vi "dfd_Render Function.vi"(0 "picture":picture, 1 "numer of element":i32=1, 3 "rect in":T1, 4 "alignment(left, top)":T2, 6 "bracket":cluster{"left":string, "right":string}={"left"="(", "right"=")"}, 7 "function name":string="y", 8 "fonts input":T3(array[cluster]), 9 "dot":bool, 11 "variable":string="n", 13 "modification":string) -> (14 "new picture":picture, 17 "rect out":T1)   [LabVIEW 2017, in "NI_DigFilter_Process.lvlib"]
uses:
  <vilib>/addons/Digital Filter Design/NI_DigFilter_Process.lvlib
panel:
  in  "Desired font(User-specified Font)":T4(ring)
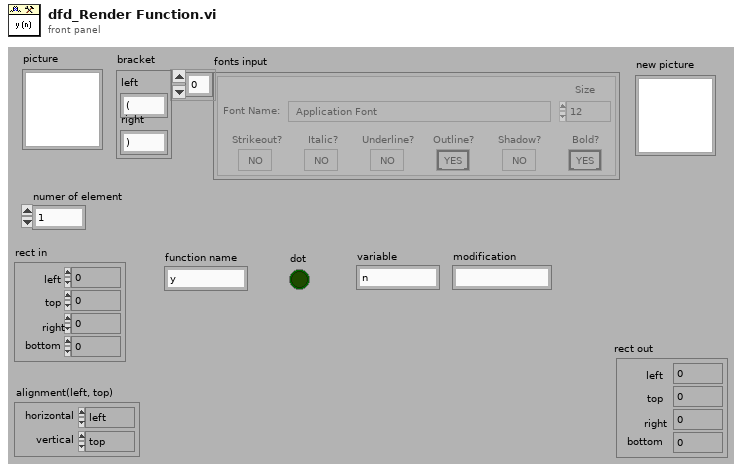
[diagram p1: front panel]
types:
  T1 = cluster{"left":i16, "top":i16, "right":i16, "bottom":i16}
  T2 = cluster{"horizontal":enum16{"left", "center", "right"}, "vertical":enum16{"top", "center", "bottom"}}
  T3 = cluster{"Font Name:":string, "Size":i16, "Strikeout?":bool, "Italic?":bool, "Underline?":bool, "Outline?":bool, "Shadow?":bool, "Bold?":bool}[]
  T4 = enum16{"User-specified Font", "Application Font", "System Font", "Dialog Font"}
  T5 = cluster{"Font Name:":string, "Size":i16, "Strikeout?":bool, "Italic?":bool, "Underline?":bool, "Outline?":bool, "Shadow?":bool, "Bold?":bool}
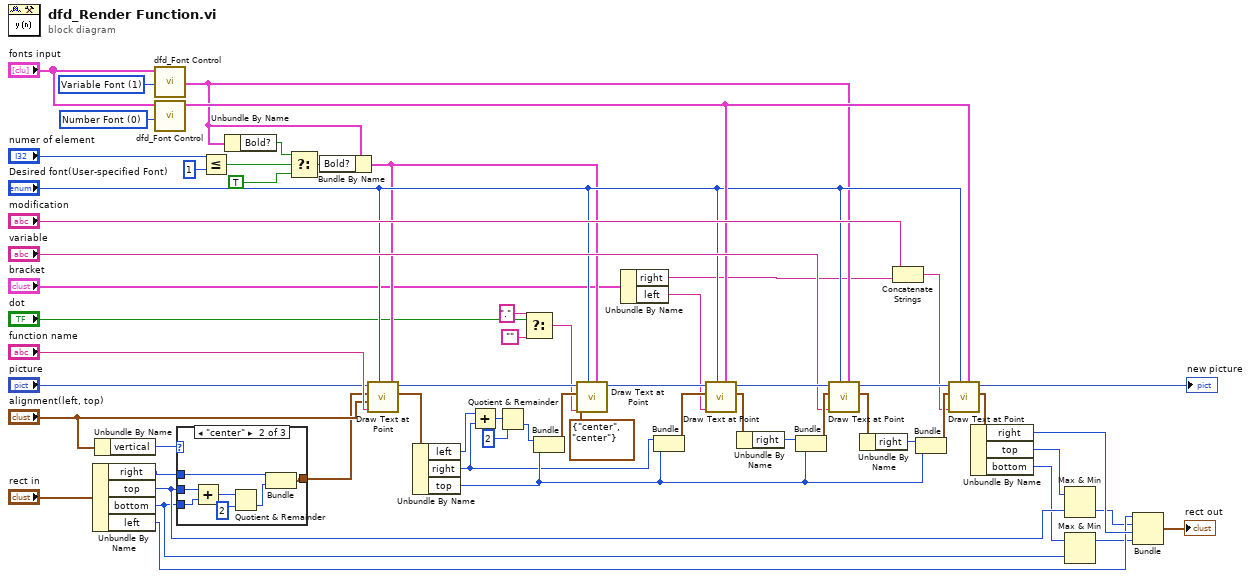
[diagram p0: block diagram]
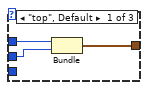
[diagram p2: hidden frame]
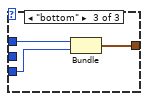
[diagram p3: hidden frame]
diagram:
  w33 = u16 1 items=["Number Font", "Variable Font", "Script Font"] ("Tpye")
  w42 = u16 0 items=["Number Font", "Variable Font", "Script Font"] ("Tpye")
  n1 = Unbundle By Name("rect in") -> ("right"=w16:i16, "top"=w12:i16, "bottom"=w5:i16, "left"=w14:i16)
  n2 = Unbundle By Name("alignment(left, top)") -> ("vertical"=w18:enum16{"top", "center", "bottom"})
  n3 = call <vilib>:"dfd_Font Control.vi"("tpye"=w33, "fonts input"="fonts input") -> ("font output"=w28:T5)  [unwired: 9 out]
  n4 = call <vilib>:"dfd_Font Control.vi"("tpye"=w42, "fonts input"="fonts input") -> ("font output"=w44:T5)  [unwired: 9 out]
  n5 = case shown="\"center\"" w18 {
    tunnel: w12 -> [w63 w70 _]
    tunnel: w16 -> [w64 w67 w74]
    tunnel: [w62 w65 w72] -> w15
    tunnel: w5 -> [_ w71 w73]
    frame "top", Default {
      n6 = Bundle("right"=w64, "top"=w63) -> (w62:cluster{"right":i16, "top":i16})  [unwired: 1 out]
    }
    frame "center" {
      n7 = Add(x=w70, y=w71) -> (x+y=w69:i16)
      n8 = Quotient & Remainder(x=w69, y=i16 2) -> (floor(x/y)=w66:i16)  [unwired: 1 out]
      n9 = Bundle("right"=w67, w66) -> (w65:cluster{"right":i16, i16})  [unwired: 1 out]
    }
    frame "bottom" {
      n10 = Bundle("right"=w74, "bottom"=w73) -> (w72:cluster{"right":i16, "bottom":i16})  [unwired: 1 out]
    }
  }
  n11 = Less Or Equal?(x="numer of element", y=1) -> (x <= y?=w41:bool)
  n12 = Unbundle By Name(w28) -> ("Bold?"=w36:bool)
  n13 = Select(t=w36, s=w41, f=TRUE) -> (s? t:f=w37:bool)
  n14 = Bundle By Name(cluster=w28, "Bold?"=w37) -> (w22:T5)
  n15 = call <vilib>:"Draw Text at Point.vi"("[user-specified font]"=w22, "desired font(Application)"="Desired font(User-specified Font)", "text"="function name", "alignment(left, top)"="alignment(left, top)", "origin"=w15, "picture"="picture") -> ("text rect"=w59:T1, "new picture"=w50:picture)  [unwired: 3 in, 1 out]
  n16 = Unbundle By Name(w59) -> ("left"=w27:i16, "right"=w26:i16, "top"=w31:i16)
  n17 = Add(x=w27, y=w26) -> (x+y=w25:i16)
  n18 = Quotient & Remainder(x=w25, y=i16 2) -> (floor(x/y)=w24:i16)  [unwired: 1 out]
  n19 = Select(t="." ("dot"), s="dot", f="") -> (s? t:f=w9:string)
  n20 = Bundle(w24, "top"=w31) -> (w35:cluster{i16, "top":i16})  [unwired: 1 out]
  n21 = call <vilib>:"Draw Text at Point.vi"("[user-specified font]"=w22, "desired font(Application)"="Desired font(User-specified Font)", "text"=w9, "alignment(left, top)"=T2 {"horizontal"=enum."center", "vertical"=enum."center"}, "origin"=w35, "picture"=w50) -> ("new picture"=w21:picture)  [unwired: 3 in, 2 out]
  n22 = Unbundle By Name("bracket") -> ("right"=w1:string, "left"=w2:string)
  n23 = Bundle("right"=w26, "top"=w31) -> (w49:cluster{"right":i16, "top":i16})  [unwired: 1 out]
  n24 = call <vilib>:"Draw Text at Point.vi"("[user-specified font]"=w44, "desired font(Application)"="Desired font(User-specified Font)", "text"=w2, "origin"=w49, "picture"=w21) -> ("text rect"=w57:T1, "new picture"=w61:picture)  [unwired: 4 in, 1 out]
  n25 = Unbundle By Name(w57) -> ("right"=w58:i16)
  n26 = Bundle("right"=w58, "top"=w31) -> (w56:cluster{"right":i16, "top":i16})  [unwired: 1 out]
  n27 = call <vilib>:"Draw Text at Point.vi"("[user-specified font]"=w28, "desired font(Application)"="Desired font(User-specified Font)", "text"="variable", "origin"=w56, "picture"=w61) -> ("text rect"=w55:T1, "new picture"=w60:picture)  [unwired: 4 in, 1 out]
  n28 = Unbundle By Name(w55) -> ("right"=w34:i16)
  n29 = Concatenate Strings("modification", w1) -> (w46:string)
  n30 = Bundle("right"=w34, "top"=w31) -> (w54:cluster{"right":i16, "top":i16})  [unwired: 1 out]
  n31 = call <vilib>:"Draw Text at Point.vi"("[user-specified font]"=w44, "desired font(Application)"="Desired font(User-specified Font)", "text"=w46, "origin"=w54, "picture"=w60) -> ("text rect"=w51:T1, "new picture"=→"new picture":picture)  [unwired: 4 in, 1 out]
  n32 = Unbundle By Name(w51) -> ("right"=w48:i16, "top"=w13:i16, "bottom"=w6:i16)
  n33 = Max & Min(x=w13, y=w12) -> (min(x,y)=w7:i16)  [unwired: 1 out]
  n34 = Max & Min(x=w6, y=w5) -> (max(x,y)=w4:i16)  [unwired: 1 out]
  n35 = Bundle("left"=w14, w7, "right"=w48, w4) -> (→"rect out":cluster{"left":i16, i16, "right":i16, i16})  [unwired: 1 out]
